vi "侦听连接请求.vi"() -> ()   [LabVIEW 2013, in "个人剂量仪-云服务器.lvclass"]
panel:
  in  "终端类型":T1(ring)
  out "队列中元素数量":i32
  in  "停止按钮":bool
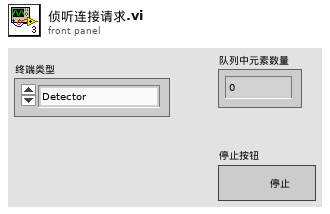
[diagram p1: front panel]
types:
  T1 = enum16{"Detector", "CenterPC", "PersonalPC", "PersonalPhone", "AdminPC"}
  T2 = enum16{"Standard", "Buffered", "CRLF", "Immediate"}
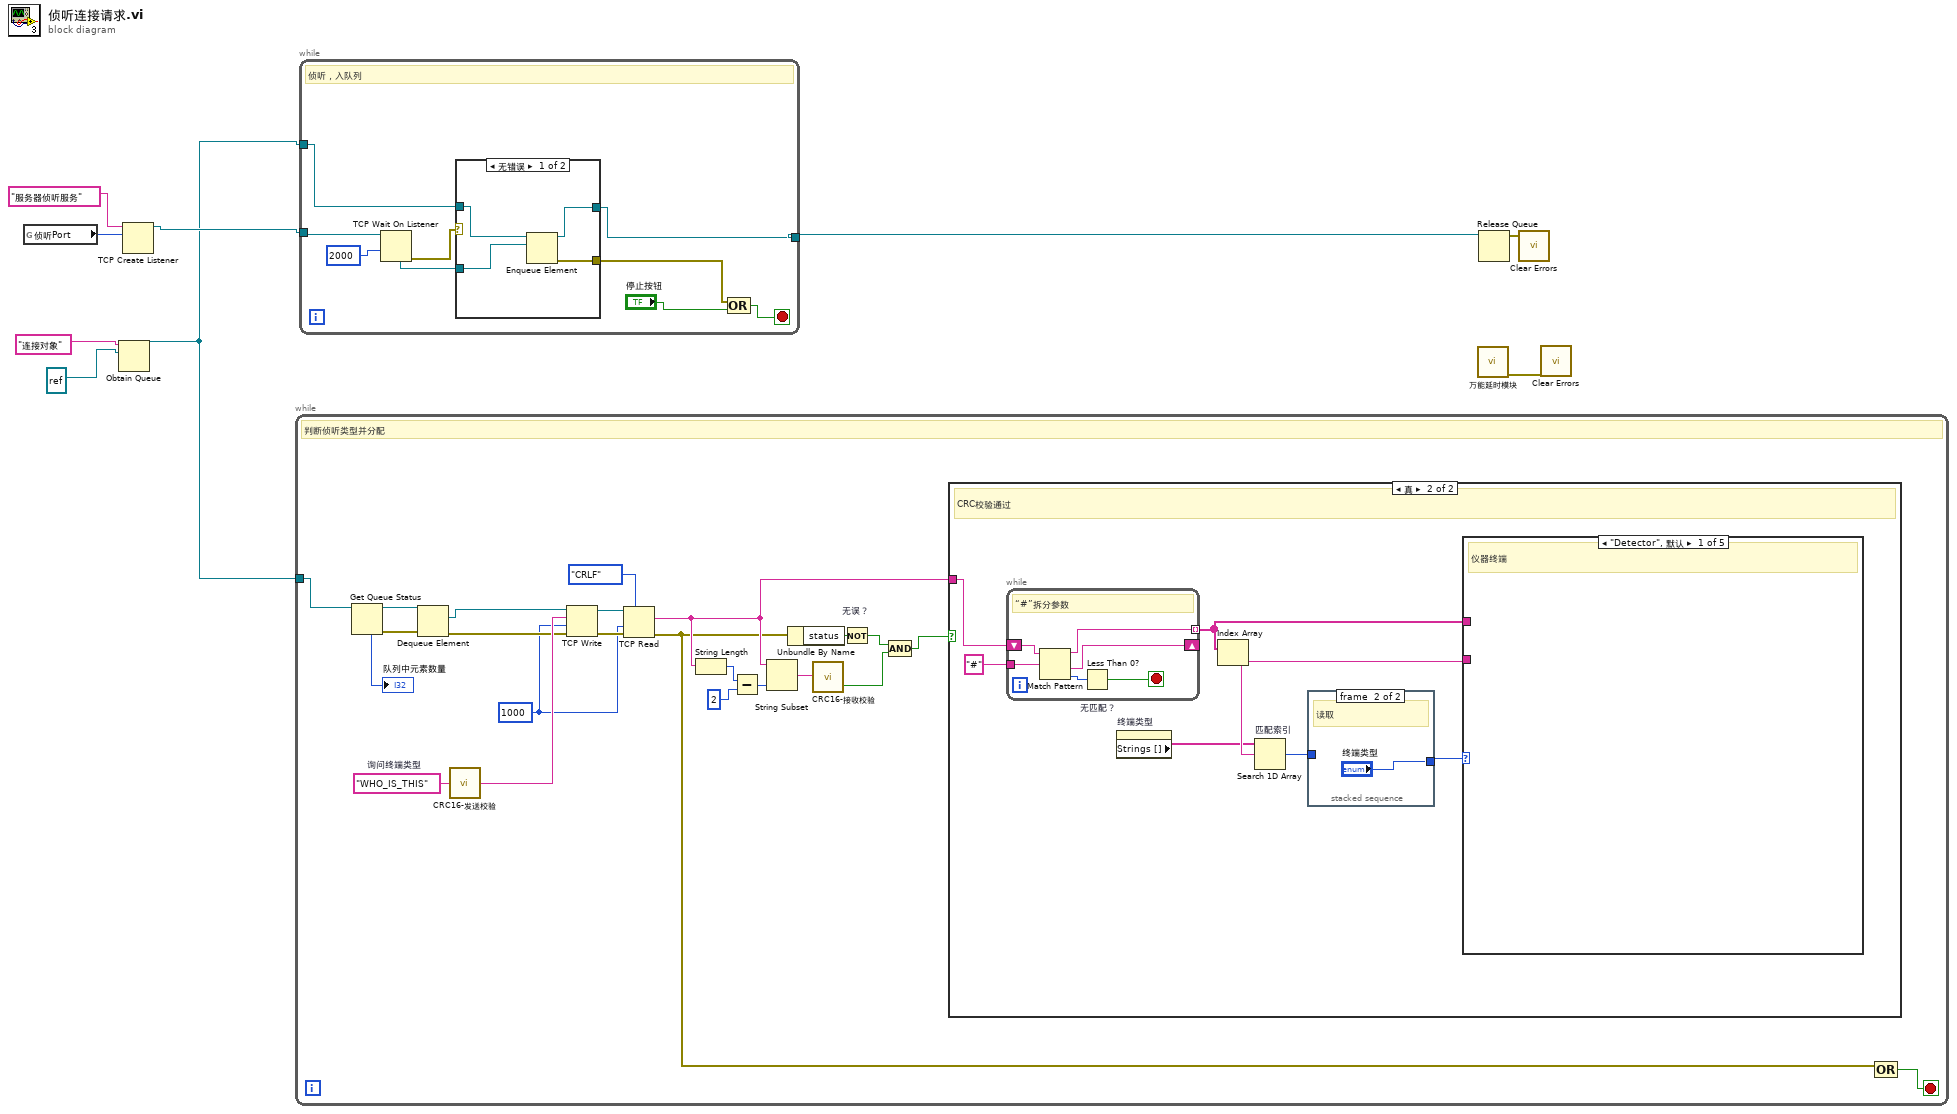
[diagram p0: block diagram]
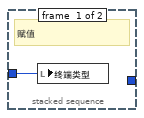
[diagram p4: hidden frame]
diagram:
  n1 = global read "server-全局变量.vi" "侦听Port"() -> (w9:u16)
  n2 = Obtain Queue(name (unnamed)="连接对象" ("名称（未命名）"), element data type=refnum<k5> refnum ("连接ID")) -> (queue out=w2:refnum<queue>)  [unwired: 3 in, 2 out]
  n3 = TCP Create Listener(10:w9, 11:"服务器侦听服务" ("服务名称")) -> (3:w6:refnum<k5>)  [unwired: 3 in, 2 out]
  n4 = while {
    tunnel: w2 -> [w30]
    stop <- w10 stop-if-true
    w22 = 1000 ("超时毫秒(25000)")
    w26 = "WHO_IS_THIS"  # 询问终端类型
    # "判断侦听类型并分配"
    n5 = Get Queue Status(queue=w30) -> (queue out=w29:refnum<queue>, error out=w32:errorcluster, # elements in queue=→"队列中元素数量":i32)  [unwired: 2 in, 5 out]
    n6 = Dequeue Element(queue=w29, error in (no error)=w32) -> (element=w24:refnum<k5>, error out=w23:errorcluster)  [unwired: 1 in, 2 out]
    n7 = call "CRC16-发送校验.vi"("净数据"=w26) -> ("完整输出"=w25:string)
    n8 = TCP Write(connection ID=w24, data in=w25, error in (no error)=w23, 9:w22) -> (connection ID out=w28:refnum<k5>, error out=w27:errorcluster)  [unwired: 1 out]
    n9 = TCP Read(connection ID=w28, error in (no error)=w27, 7:T2."CRLF" ("模式（标准）"), 9:w22) -> (data out=w12:string, error out=w11:errorcluster)  [unwired: 1 in, 1 out]
    n10 = String Length(string=w12) -> (length=w20:i32)
    n11 = Subtract(x=w20, y=2 ("x")) -> (x-y=w18:i32)
    n12 = String Subset(string=w12, length (rest)=w18) -> (substring=w17:string)  [unwired: 1 in]
    n13 = Unbundle By Name(w11) -> ("status"=w14:bool)
    n14 = call "CRC16-接收校验.vi"("读取缓冲区"=w17) -> ("CRC？"=w16:bool)  [unwired: 1 out]
    n15 = Not "无误？"(x=w14) -> (.not. x?=w13:bool)
    n16 = Compound Arithmetic op=AND(w13, w16) -> (w15:bool)
    n17 = case shown="真" w15 {
      tunnel: w12 -> [_ w37]
      frame False {
      }
      frame True {
        # "CRC校验通过"
        n18 = while {
          tunnel: "#" ("正则表达式") -> [w44]
          shift-right: [w43] -> _
          shift-left: w37 -> [w45]
          tunnel: [w42] -> w35 mode=indexing
          stop <- w40 stop-if-true
          # "“#”拆分参数"
          n19 = Match Pattern ("终端类型")(string=w45, regular expression=w44) -> (before substring=w42:string, after substring=w43:string, offset past match=w41:i32)  [unwired: 1 in, 1 out]
          n20 = Less Than 0? "无匹配？"(x=w41) -> (x < 0?=w40:bool)
        }
        n21 = property on="终端类型" class="Enum (严格)"() -> ("Strings []"=w33:string[])  [unwired: 2 in, 2 out]
        n22 = Index Array(array=w35) -> (element=w34:string)  [unwired: 1 in]
        n23 = Search 1D Array "匹配索引"(1D array=w33, element=w34) -> (index of element=w39:i32)  [unwired: 1 in]
        n24 = stacked-sequence {
          tunnel: w39 -> [w46 _]
          tunnel: [_ "终端类型"] -> w38
          frame #0 {
            # "赋值"
            n25 = local write "终端类型"(w46) -> ()
          }
          frame #1 {
            # "读取"
          }
        }
        n26 = case shown="\"Detector\", 默认" w38 {
          tunnel: w34 -> [_ _ _ _ _]
          tunnel: w35 -> [_ _ _ _ _]
          frame "Detector", Default {
            # "仪器终端"
          }
          frame "CenterPC" {
            # "PC总上位机"
          }
          frame "PersonalPC" {
            # "PC个人上位机"
          }
          frame "PersonalPhone" {
            # "手机个人上位机"
          }
          frame "AdminPC" {
            # "服务器管理员客户端"
          }
        }
      }
    }
    n27 = Compound Arithmetic op=OR(w11) -> (w10:bool)  [unwired: 1 in]
  }
  n28 = while {
    tunnel: w6 -> [w56]
    tunnel: w2 -> [w52]
    tunnel: [w48] -> w3
    stop <- w49 stop-if-true
    # "侦听，入队列"
    n29 = TCP Wait On Listener(9:2000 ("超时毫秒（一直等待:-1）"), 11:w56) -> (0:w54:errorcluster, 4:w53:refnum<k5>)  [unwired: 2 in, 3 out]
    n30 = case shown="无错误" w54 {
      tunnel: w53 -> [w60 _]
      tunnel: w52 -> [w59 w61]
      tunnel: [w58 _] -> w51
      tunnel: [w57 w61] -> w48
      frame No Error {
        n31 = Enqueue Element(queue=w59, element=w60) -> (queue out=w57:refnum<queue>, error out=w58:errorcluster)  [unwired: 2 in, 1 out]
      }
      frame Error {
      }
    }
    n32 = Compound Arithmetic op=OR(w51, "停止按钮") -> (w49:bool)
  }
  n33 = call "万能延时模块.vi"() -> ("错误输出"=w1:errorcluster)  [unwired: 10 in, 1 out]
  n34 = Release Queue(queue=w3) -> (error out=w4:errorcluster)  [unwired: 2 in, 2 out]
  n35 = call <vilib>:"Clear Errors.vi"("error in (no error)"=w4) -> ()  [unwired: 6 in, 1 out]
  n36 = call <vilib>:"Clear Errors.vi"("error in (no error)"=w1) -> ()  [unwired: 6 in, 1 out]
